vi "串口调试程序.VI"() -> ()   [LabVIEW 2017]
uses:
  <vilib>/Instr/_visa.llb/VISA Configure Serial Port (Instr).vi
panel:
  out "当前时间":timestamp
  in  "清零":bool
  out "接收字节数":u32
  out "发送字节数":u32
  in  "Boolean 9":bool
  in  "毫秒倍数":u32=100 min=2 step=1
  in  "自动发送":bool
  in  "十六进制发送":bool
  in  "OK Button 2":bool
  in  "十六进制接收":bool
  in  "Boolean 8":bool
  in  "退出":bool
  out "接收数据区：":string
  in  "发送数据区：":string="作者:3243825512@qq.com"
  in  "发送":bool
  in  "打开":bool caption="stop"
  in  "校验位：":u16(ring) items=["  无校验", "  奇校验", "  偶校验"]
  in  "波特率：":u16(ring)=11 items=["   300", "   600", "   1200", "   2400", "   4800   ", "   9600", "   19200", "   38400", "   43000", "   56000", "   57600", "   115200"]
  in  "通讯口：":u16(ring) items=["   com1", "   com2", "   com3", "   com4", "   com5"]
  # "通讯口设置："
  # "接收数据设置："
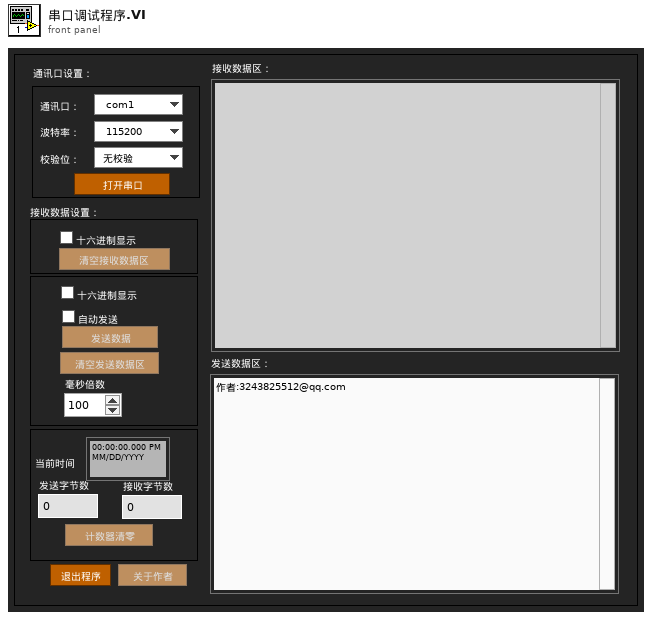
[diagram p1: front panel]
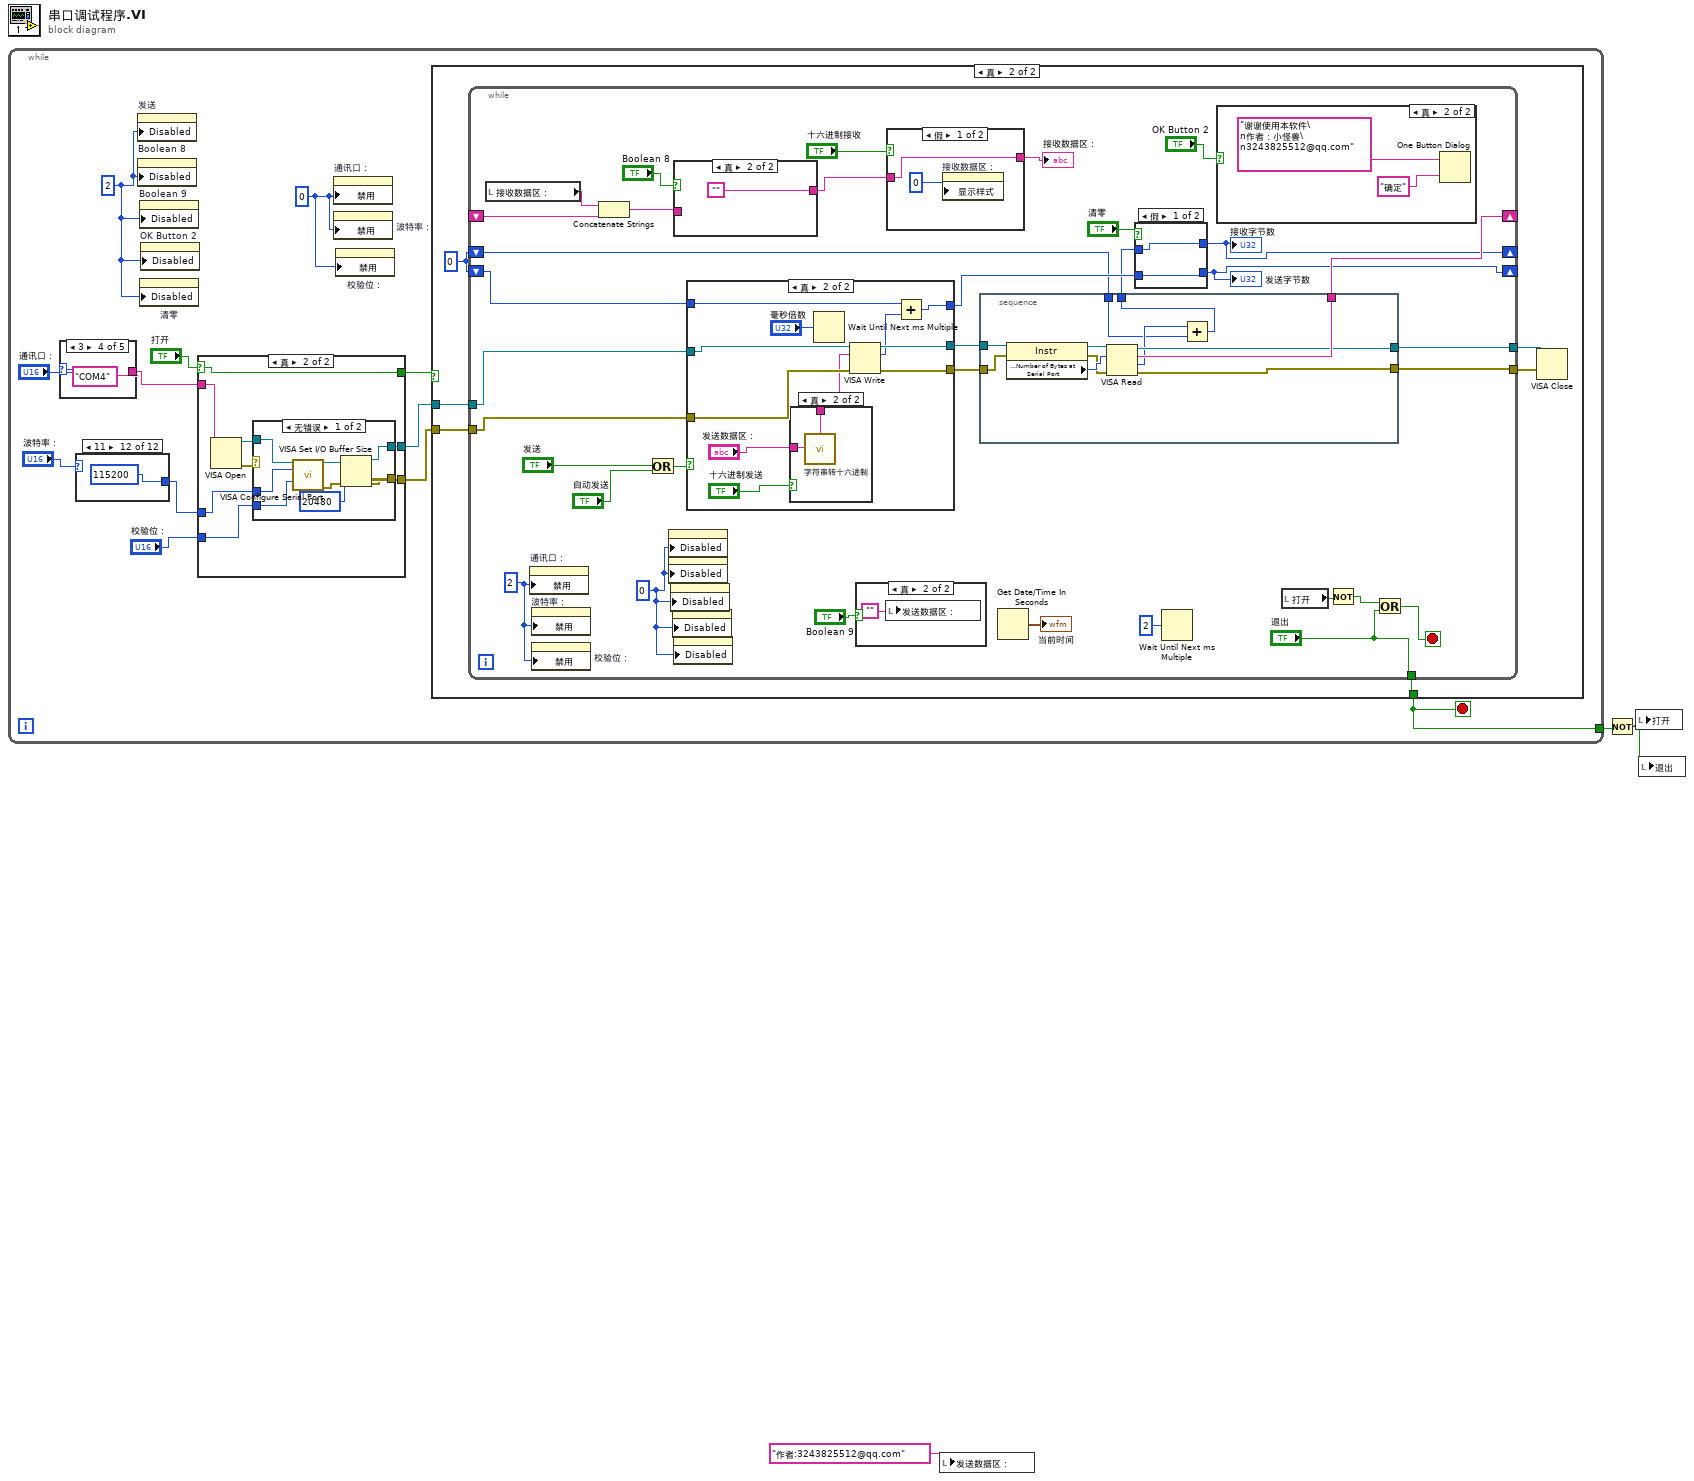
[diagram p0: block diagram]
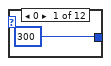
[diagram p2: hidden frame]
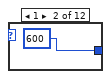
[diagram p3: hidden frame]
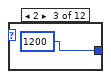
[diagram p4: hidden frame]
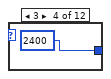
[diagram p5: hidden frame]
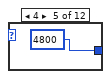
[diagram p6: hidden frame]
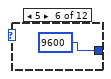
[diagram p7: hidden frame]
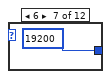
[diagram p8: hidden frame]
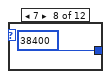
[diagram p9: hidden frame]
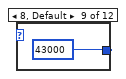
[diagram p10: hidden frame]
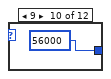
[diagram p11: hidden frame]
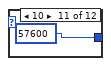
[diagram p12: hidden frame]
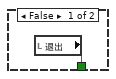
[diagram p13: hidden frame]
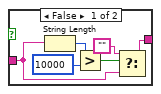
[diagram p14: hidden frame]
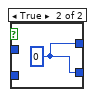
[diagram p15: hidden frame]
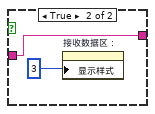
[diagram p20: hidden frame]
diagram:
  n1 = while {
    tunnel: [w8] -> w3
    stop <- w8 stop-if-true
    w6 = 2
    w10 = 0
    n2 = case shown="3" "通讯口：" {
      tunnel: ["COM1" "COM2" "COM3" "COM4" "COM5"] -> w9
      frame 0, Default {
      }
      frame 1 {
      }
      frame 2 {
      }
      frame 3 {
      }
      frame 4 {
      }
    }
    n3 = case shown="11" "波特率：" {
      tunnel: [300 600 1200 2400 4800 9600 19200 38400 43000 56000 57600 115200] -> w4
      frame 0 {
      }
      frame 1 {
      }
      frame 2 {
      }
      frame 3 {
      }
      frame 4 {
      }
      frame 5 {
      }
      frame 6 {
      }
      frame 7 {
      }
      frame 8, Default {
      }
      frame 9 {
      }
      frame 10 {
      }
      frame 11 {
      }
    }
    n4 = property on="发送" class="Bool"("Disabled"=w6) -> ()  [unwired: 2 in, 2 out]
    n5 = property on="Boolean 8" class="Bool"("Disabled"=w6) -> ()  [unwired: 2 in, 2 out]
    n6 = property on="Boolean 9" class="Bool"("Disabled"=w6) -> ()  [unwired: 2 in, 2 out]
    n7 = property on="清零" class="Bool"("Disabled"=w6) -> ()  [unwired: 2 in, 2 out]
    n8 = property on="OK Button 2" class="Bool"("Disabled"=w6) -> ()  [unwired: 2 in, 2 out]
    n9 = case shown="真" "打开" {
      selector: "打开" -> [w114 w122]
      tunnel: w4 -> [_ w118]
      tunnel: [w114 w122] -> w13
      tunnel: [_ w116] -> w12
      tunnel: [_ w115] -> w11
      tunnel: w9 -> [_ w121]
      tunnel: "校验位：" -> [_ w117]
      frame False {
      }
      frame True {
        n10 = VISA Open(VISA resource name=w121) -> (VISA resource name=w119:refnum<visa-resource-name>, error out=w120:errorcluster)  [unwired: 4 in]
        n11 = case shown="无错误" w120 {
          tunnel: w119 -> [w130 _]
          tunnel: w118 -> [w129 _]
          tunnel: w117 -> [w128 _]
          tunnel: [w124 _] -> w116
          tunnel: [w125 _] -> w115
          frame No Error {
            n12 = call-poly "VISA Configure Serial Port"("VISA resource name"=w130, "baud rate (9600)"=w129, "parity (0:none)"=w128) -> ("VISA resource name out"=w127:refnum<visa-resource-name>, "error out"=w126:errorcluster)  [unwired: 11 in]
            n13 = VISA Set I/O Buffer Size(VISA resource name=w127, size (4096)=u32 20480 ("大小(4096)"), error in (no error)=w126) -> (VISA resource name out=w124:refnum<visa-resource-name>, error out=w125:errorcluster)  [unwired: 1 in]
          }
          frame Error {
            n14 = One Button Dialog(message="ERROR!" ("消息")) -> ()  [unwired: 1 in, 1 out]
          }
        }
      }
    }
    n15 = property on="通讯口：" class="Ring (严格)"("禁用"=w10) -> ()  [unwired: 2 in, 2 out]
    n16 = property on="波特率：" class="Ring (严格)"("禁用"=w10) -> ()  [unwired: 2 in, 2 out]
    n17 = property on="校验位：" class="Ring (严格)"("禁用"=w10) -> ()  [unwired: 2 in, 2 out]
    n18 = case shown="真" w13 {
      tunnel: w12 -> [_ w34]
      tunnel: w11 -> [_ w33]
      tunnel: [w28 w30] -> w8
      frame False {
        n19 = local read "退出"() -> (w28:bool)
      }
      frame True {
        w29 = 0
        n20 = while {
          shift-right: [w68] -> _
          shift-left: _ -> [w66]
          tunnel: w34 -> [w62]
          tunnel: w33 -> [w61]
          tunnel: ["退出"] -> w30
          tunnel: [w55] -> w32
          tunnel: [w54] -> w31
          shift-right: [w40] -> _
          shift-left: w29 -> [w38]
          shift-right: [w39] -> _
          shift-left: w29 -> [w41]
          stop <- w52 stop-if-true
          w43 = 0
          w60 = 2
          n21 = local read "接收数据区："() -> (w67:string)
          n22 = property on="通讯口：" class="Ring (严格)"("禁用"=w60) -> ()  [unwired: 2 in, 2 out]
          n23 = property on="波特率：" class="Ring (严格)"("禁用"=w60) -> ()  [unwired: 2 in, 2 out]
          n24 = property on="校验位：" class="Ring (严格)"("禁用"=w60) -> ()  [unwired: 2 in, 2 out]
          n25 = Concatenate Strings(w67, w66) -> (w36:string)
          n26 = Or(x="发送", y="自动发送") -> (x .or. y?=w56:bool)
          n27 = property on="发送" class="Bool"("Disabled"=w43) -> ()  [unwired: 2 in, 2 out]
          n28 = property on="Boolean 8" class="Bool"("Disabled"=w43) -> ()  [unwired: 2 in, 2 out]
          n29 = property on="Boolean 9" class="Bool"("Disabled"=w43) -> ()  [unwired: 2 in, 2 out]
          n30 = property on="OK Button 2" class="Bool"("Disabled"=w43) -> ()  [unwired: 2 in, 2 out]
          n31 = case shown="真" "Boolean 8" {
            tunnel: [w70 ""] -> w35
            tunnel: w36 -> [w71 _]
            frame False {
              n32 = String Length(string=w71) -> (length=w74:i32)
              n33 = Greater?(x=w74, y=10000) -> (0:w72:bool)
              n34 = Select(t="", s=w72, f=w71) -> (s? t:f=w70:string)
            }
            frame True {
            }
          }
          n35 = property on="清零" class="Bool"("Disabled"=w43) -> ()  [unwired: 2 in, 2 out]
          n36 = case shown="真" w56 {
            tunnel: w62 -> [w93 w104]
            tunnel: w61 -> [w92 w103]
            tunnel: [w93 w102] -> w59
            tunnel: [w92 w101] -> w58
            tunnel: w41 -> [w91 w95]
            tunnel: [w91 w94] -> w45
            frame False {
            }
            frame True {
              n37 = case shown="真" "十六进制发送" {
                tunnel: "发送数据区：" -> [w105 w107]
                tunnel: [w105 w106] -> w99
                frame False {
                }
                frame True {
                  n38 = call "字符串转十六进制.vi"("字符串"=w107) -> ("十六进制整型字符串"=w106:string)  [unwired: 10 in]
                }
              }
              n39 = Wait Until Next ms Multiple(millisecond multiple="毫秒倍数") -> ()  [unwired: 1 out]
              n40 = VISA Write(VISA resource name=w104, write buffer=w99, error in (no error)=w103) -> (VISA resource name out=w102:refnum<visa-resource-name>, return count=w96:u32, error out=w101:errorcluster)
              n41 = Add(x=w95, y=w96) -> (x+y=w94:u32)
            }
          }
          n42 = case shown="真" "Boolean 9" {
            frame False {
            }
            frame True {
              n43 = local write "发送数据区："("") -> ()
            }
          }
          n44 = case shown="假" "十六进制接收" {
            tunnel: [w110 w112] -> w64
            tunnel: w35 -> [w110 w112]
            frame False {
              n45 = property on="接收数据区：" class="Str"("显示样式"=0) -> ()  [unwired: 2 in, 2 out]
            }
            frame True {
              n46 = property on="接收数据区：" class="Str"("显示样式"=3) -> ()  [unwired: 2 in, 2 out]
            }
          }
          "接收数据区：" <- w64
          n47 = stacked-sequence {
            tunnel: w59 -> [w90]
            tunnel: w58 -> [w87]
            tunnel: [w85] -> w68
            tunnel: [w84] -> w55
            tunnel: [w81] -> w54
            tunnel: [w82] -> w44
            tunnel: w38 -> [w80]
            frame #0 {
              n48 = property class="Instr"(reference=w90, error in=w87) -> (reference out=w88:refnum<visa-resource-name>, error out=w86:errorcluster, "Serial Settings:Number of Bytes at Serial Port"=w89:u32)
              n49 = VISA Read(VISA resource name=w88, byte count=w89, error in (no error)=w86) -> (VISA resource name out=w84:refnum<visa-resource-name>, read buffer=w85:string, return count=w83:u32, error out=w81:errorcluster)
              n50 = Add(x=w83, y=w80) -> (x+y=w82:u32)
            }
          }
          n51 = Get Date/Time In Seconds() -> (seconds since 1Jan1904=→"当前时间":timestamp)
          n52 = case shown="假" "清零" {
            tunnel: [w77 w78] -> w39
            tunnel: w45 -> [w77 _]
            tunnel: w44 -> [w76 _]
            tunnel: [w76 w78] -> w40
            frame False {
            }
            frame True {
              w78 = 0
            }
          }
          "发送字节数" <- w39
          "接收字节数" <- w40
          n53 = Wait Until Next ms Multiple(millisecond multiple=u32 2 ("毫秒倍数")) -> ()  [unwired: 1 out]
          n54 = case shown="真" "OK Button 2" {
            frame False {
            }
            frame True {
              n55 = One Button Dialog(message="谢谢使用本软件\n作者：小怪兽\n3243825512@qq.com", button name ("OK")="确定") -> ()  [unwired: 1 out]
            }
          }
          n56 = local read "打开"() -> (w50:bool)
          n57 = Not(x=w50) -> (.not. x?=w49:bool)
          n58 = Or(x=w49, y="退出") -> (x .or. y?=w52:bool)
        }
        n59 = VISA Close(VISA resource name=w32, error in (no error)=w31) -> ()  [unwired: 1 out]
      }
    }
  }
  n60 = local write "发送数据区："("作者:3243825512@qq.com" ("发送数据区：")) -> ()
  n61 = Not(x=w3) -> (.not. x?=w2:bool)
  n62 = local write "打开"(w2) -> ()
  n63 = local write "退出"(w2) -> ()
